vi "Lifter PID.vi"(11 "MechanismMetrics in":T1={"lift height"=1500.0, "Command"=enum."Noop", "Time Stamp"=0, "ToggleCollector"=FALSE, "Bottom_Limit_Switch "=FALSE, "Top_Limit_Switch"=FALSE, "lift power"=0.0, "Elevator soleniod debounce time   "=0.0, "LifterOverride"=FALSE, "Previous Lift power"=0.0, "manual lift"=0.0, "Lifter State"=enum."LifterOpen", "Auto Lifter State"=enum."Not Pressed", "Toggle Auto Lifter"=FALSE, "Wait Timer"=0.0, "HP Auto Indexer"=FALSE, "HP Auto Lifter State"=enum."Not Pressed"}) -> (0 "MechanismMetrics in 2":T1={"lift height"=1500.0, "Command"=enum."Noop", "Time Stamp"=0, "ToggleCollector"=FALSE, "Bottom_Limit_Switch "=FALSE, "Top_Limit_Switch"=FALSE, "lift power"=0.0, "Elevator soleniod debounce time   "=0.0, "LifterOverride"=FALSE, "Previous Lift power"=0.0, "manual lift"=0.0, "Lifter State"=enum."LifterOpen", "Auto Lifter State"=enum."Not Pressed", "Toggle Auto Lifter"=FALSE, "Wait Timer"=0.0, "HP Auto Indexer"=FALSE, "HP Auto Lifter State"=enum."Not Pressed"})   [LabVIEW 2014]
uses:
  MechanismMetrics.ctl
  Lifter States.ctl
  Auto Lifter States.ctl
  encoderData.vi
  <vilib>/addons/control/pid/pid.llb/PID (DBL).vi
  <vilib>/addons/control/pid/NI_PID_pid.lvlib
panel:
  in  "output low":dbl
  in  "output high":dbl=0.25
  in  "derivative time (Td, min)":dbl
  in  "integral time (Ti, min)":dbl
  in  "proportional gain (Kc)":dbl=0.01
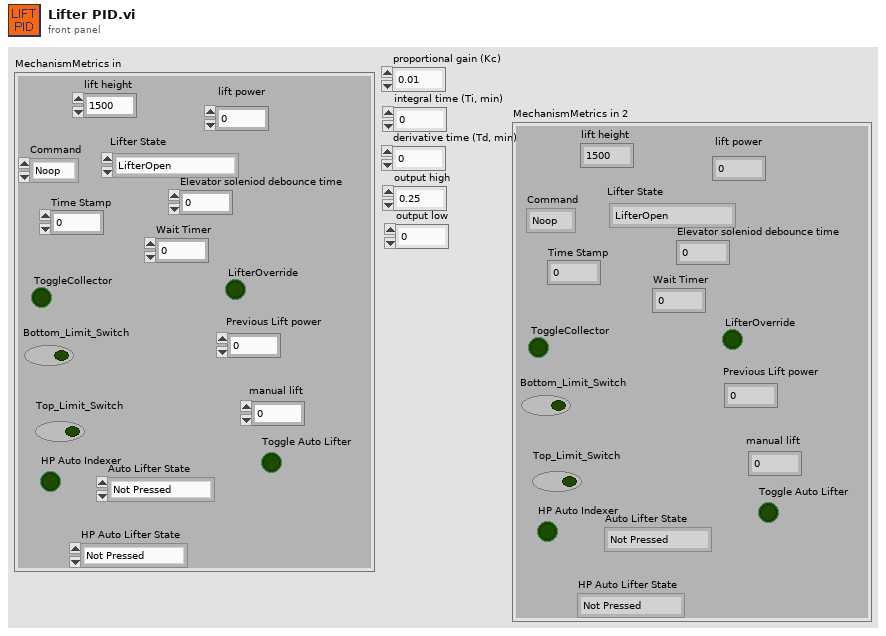
[diagram p1: front panel]
types:
  T1 = typedef "MechanismMetrics.ctl" = cluster{"lift height":dbl, "Command":enum16{"Noop", "Flagged"}, "Time Stamp":u32, "ToggleCollector":bool, "Bottom_Limit_Switch ":bool, "Top_Limit_Switch":bool, "lift power":dbl, "Elevator soleniod debounce time   ":dbl, "LifterOverride":bool, "Previous Lift power":dbl, "manual lift":dbl, "Lifter State":T2, "Auto Lifter State":T3, "Toggle Auto Lifter":bool, "Wait Timer":dbl, "HP Auto Indexer":bool, "HP Auto Lifter State":T3}
  T2 = typedef "Lifter States.ctl" = enum16{"OpeningLifter", "LifterOpen", "ClosingLifter", "LifterClosed"}
  T3 = typedef "Auto Lifter States.ctl" = enum16{"Not Pressed", "THE_END", "WAIT_FOR_RELEASE", "Press Detected", "To Release Stacked1", "To Collect", "Open Lifter", "WAIT", "Close", "To Stack1"}
  T4 = cluster{"proportional gain (Kc)":dbl, "integral time (Ti, min)":dbl, "derivative time (Td, min)":dbl}
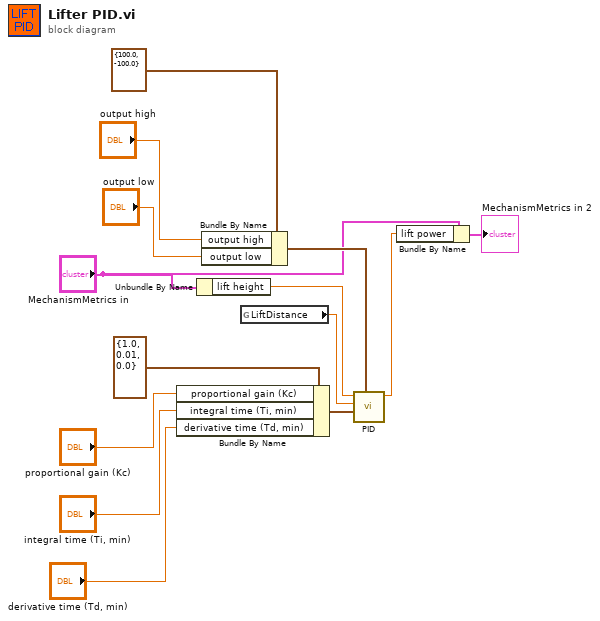
[diagram p0: block diagram]
diagram:
  n1 = Bundle By Name(cluster=T4 {"proportional gain (Kc)"=1.0, "integral time (Ti, min)"=0.01, "derivative time (Td, min)"=0.0} ("PID gains"), "proportional gain (Kc)"="proportional gain (Kc)", "integral time (Ti, min)"="integral time (Ti, min)", "derivative time (Td, min)"="derivative time (Td, min)") -> (w11:T4)
  n2 = Unbundle By Name("MechanismMetrics in") -> ("lift height"=w14:dbl)
  n3 = Bundle By Name(cluster=cluster{"output high":dbl, "output low":dbl} {"output high"=100.0, "output low"=-100.0} ("output range"), "output high"="output high", "output low"="output low") -> (w9:cluster{"output high":dbl, "output low":dbl})
  n4 = global read "encoderData.vi" "LiftDistance"() -> (w13:dbl)
  n5 = call-poly <vilib>:"PID.vi"("output range"=w9, "PID gains"=w11, "process variable"=w13, "setpoint"=w14) -> ("output"=w2:dbl)  [unwired: 6 in, 1 out]
  n6 = Bundle By Name(cluster="MechanismMetrics in", "lift power"=w2) -> (→"MechanismMetrics in 2":T1)
